vi "Defaults.vi"() -> (2 "Defaults":T1)   [LabVIEW 2020, in "VolatusGUIElements.lvlib" / "DigitalButtonControl.lvclass"]
uses:
  DigitalButtonControl.lvclass
  DigitalButtonControl.lvclass/DigitalButtonControl.ctl
  Appearance.ctl
  JSON.ctl
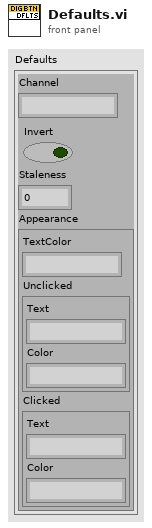
[diagram p1: front panel]
types:
  T1 = typedef "VolatusGUIElements.lvlib/DigitalButtonControl.lvclass/JSON.ctl" = cluster{"Channel":string, "Invert":bool, "Staleness":dbl, "Appearance":cluster{"TextColor":string, "Unclicked":T2, "Clicked":T2}}
  T2 = typedef "VolatusGUIElements.lvlib/DigitalButtonControl.lvclass/Appearance.ctl" = cluster{"Text":string, "Color":string}
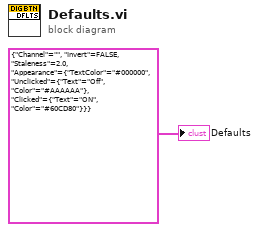
[diagram p0: block diagram]
diagram:
  "Defaults" <- T1 {"Channel"="", "Invert"=FALSE, "Staleness"=2.0, "Appearance"={"TextColor"="#000000", "Unclicked"={"Text"="Off", "Color"="#AAAAAA"}, "Clicked"={"Text"="ON", "Color"="#60CD80"}}} ("JSON")
